vi "Take_PicV2.vi"(10 "Image Src":T1, 11 "CameraDevRef":T2) -> (3 "Image Out":T1)   [LabVIEW 2011]
uses:
  <vilib>/Rock Robotics/WPI/Camera/WPI_CameraDevRef.ctl
  <vilib>/vision/Image Controls.llb/IMAQ Image.ctl
  <vilib>/Rock Robotics/WPI/Relay/WPI_RelayValue.ctl
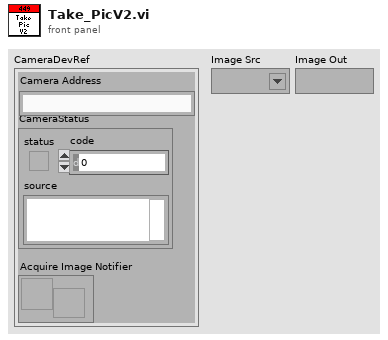
[diagram p1: front panel]
types:
  T1 = typedef "IMAQ Image.ctl" = refnum<image>
  T2 = typedef "WPI_CameraDevRef.ctl" = cluster{"Camera Address":string, "CameraStatus":errorcluster, "Acquire Image Notifier":refnum<notifier>}
  T3 = typedef "WPI_RelayValue.ctl" = enum16{"Off", "On", "Forward", "Reverse"}
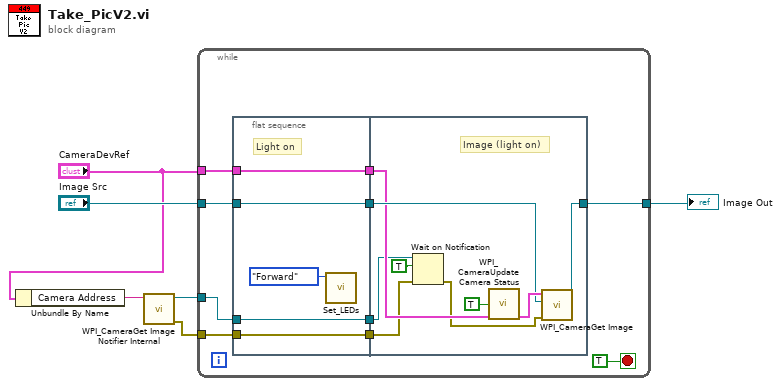
[diagram p0: block diagram]
diagram:
  n1 = Unbundle By Name("CameraDevRef") -> ("Camera Address"=w4:string)
  n2 = call <vilib>:"WPI_CameraGet Image Notifier Internal.vi"("Camera Address"=w4) -> ("error out"=w1:errorcluster, "Image Notifier"=w2:refnum<notifier>)  [unwired: 9 in]
  n3 = while {
    tunnel: "CameraDevRef" -> [w16]
    tunnel: "Image Src" -> [w15]
    tunnel: [w13] -> w5
    tunnel: w2 -> [w12]
    tunnel: w1 -> [w11]
    stop <- TRUE stop-if-true
    n4 = flat-sequence {
      tunnel: w16 -> [w20]
      tunnel: w15 -> [w19]
      tunnel: [w20] -> w10
      tunnel: [w19] -> w9
      tunnel: w12 -> [w18]
      tunnel: [w18] -> w8
      tunnel: [w17] -> w7
      tunnel: w11 -> [w17]
      tunnel: w10 -> [w26]
      tunnel: w9 -> [w28]
      tunnel: w8 -> [w22]
      tunnel: w7 -> [w24]
      tunnel: [w27] -> w13
      frame #0 {
        # "Light on"
        n5 = call "Set_LEDs.vi"("RelayValue"=WPI_RelayValue."Forward") -> ()  [unwired: 10 in, 1 out]
      }
      frame #1 {
        # "Image (light on)"
        n6 = Wait on Notification(notifier=w22, ignore previous (F)=TRUE, error in (no error)=w24) -> (error out=w23:errorcluster)  [unwired: 1 in, 3 out]
        n7 = call <vilib>:"WPI_CameraUpdate Camera Status.vi"("CameraDevRef In"=w26, "Enable Vision"=TRUE) -> ("CameraDevRef Out"=w30:T2)  [unwired: 3 in]
        n8 = call <vilib>:"WPI_CameraGet Image.vi"("error in (no error)"=w23, "Image"=w28, "CameraDevRef"=w30) -> ("Image Out"=w27:T1)  [unwired: 6 in, 2 out]
      }
    }
  }
  "Image Out" <- w5
